vi "Begin.vi"() -> (0 "Error Out":errorcluster)   [LabVIEW 2020]
doc: "This VI opens device references, sets constants, clears hardware sticky faults, defines static VI references, and resets gobal variables."
uses:
  <vilib>/Rock Robotics/WPI/DriverStation/WPI_DriverStationRobotMode2.ctl
  driverdata.vi
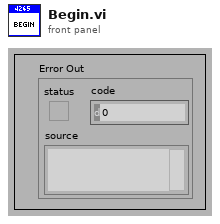
[diagram p1: front panel]
types:
  T1 = typedef "WPI_DriverStationRobotMode2.ctl" = enum16{"Autonomous Disabled", "Autonomous Enabled", "Teleop Disabled", "Teleop Enabled", "Disconnected", "Finish", "Test Disabled", "Test Enabled", "Emergency Stopped"}
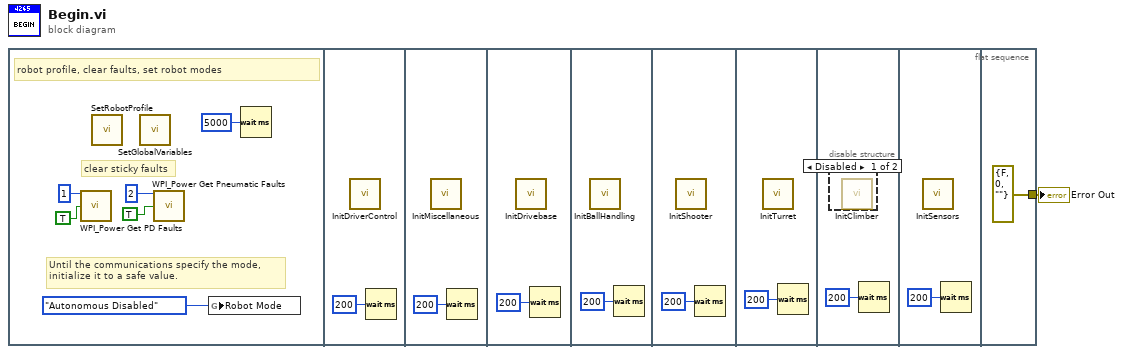
[diagram p0: block diagram]
diagram:
  n1 = flat-sequence {
    tunnel: [errorcluster {"status"=FALSE, "code"=0, "source"=""} ("error in")] -> w1
    frame #0 {
      # "clear sticky faults"
      # "Until the communications specify the mode,\ninitialize it to a safe value."
      # "robot profile, clear faults, set robot modes"
      n2 = call <vilib>:"WPI_Power Get PD Faults.vi"("Power Distribution (def)"=u8 1 ("Power Distribution Panel (0)"), "Clear Sticky Faults"=TRUE) -> ()  [unwired: 10 in, 4 out]
      n3 = call "SetRobotProfile.vi"() -> ()  [unwired: 1 in]
      n4 = call "SetGlobalVariables.vi"() -> ()  [unwired: 1 in]
      n5 = call <vilib>:"WPI_Power Get Pneumatic Faults.vi"("Pneumatics device (def)"=u8 2 ("Pneumatics Control Module (0)"), "Clear Sticky Faults"=TRUE) -> ()  [unwired: 8 in, 6 out]
      n6 = global write "driverdata.vi" "Robot Mode"(WPI_DriverStationRobotMode2."Autonomous Disabled" ("Robot Mode")) -> ()
      n7 = Wait (ms)(milliseconds to wait=u32 5000) -> ()  [unwired: 1 out]
    }
    frame #1 {
      n8 = call "InitDriverControl.vi"() -> ()  [unwired: 12 in]
      n9 = Wait (ms)(milliseconds to wait=u32 200) -> ()  [unwired: 1 out]
    }
    frame #2 {
      n10 = call "InitMiscellaneous.vi"() -> ()  [unwired: 12 in]
      n11 = Wait (ms)(milliseconds to wait=u32 200) -> ()  [unwired: 1 out]
    }
    frame #3 {
      n12 = call "InitDrivebase.vi"() -> ()  [unwired: 1 in]
      n13 = Wait (ms)(milliseconds to wait=u32 200) -> ()  [unwired: 1 out]
    }
    frame #4 {
      n14 = call "InitBallHandling.vi"() -> ()  [unwired: 1 in]
      n15 = Wait (ms)(milliseconds to wait=u32 200) -> ()  [unwired: 1 out]
    }
    frame #5 {
      n16 = call "InitShooter.vi"() -> ()  [unwired: 1 in]
      n17 = Wait (ms)(milliseconds to wait=u32 200) -> ()  [unwired: 1 out]
    }
    frame #6 {
      n18 = call "InitTurret.vi"() -> ()  [unwired: 1 in]
      n19 = Wait (ms)(milliseconds to wait=u32 200) -> ()  [unwired: 1 out]
    }
    frame #7 {
      n20 = disable-structure shown="Disabled" {
        frame Disabled {
          n21 = call "InitClimber.vi"() -> ()  [unwired: 1 in]
        }
        frame Enabled {
        }
      }
      n22 = Wait (ms)(milliseconds to wait=u32 200) -> ()  [unwired: 1 out]
    }
    frame #8 {
      n23 = call "InitSensors.vi"() -> ()  [unwired: 1 in]
      n24 = Wait (ms)(milliseconds to wait=u32 200) -> ()  [unwired: 1 out]
    }
    frame #9 {
    }
  }
  "Error Out" <- w1
